vi "4_6.vi"() -> ()   [LabVIEW 2020]
uses:
  <vilib>/numeric/Random Number (Range) U64.vi
  <vilib>/numeric/sub_Random U32.vi
panel:
  in  "Numeric":i32
  out "nieparzyste":u64[](array[numeric])
  out "parzyste":u64[](array[numeric])
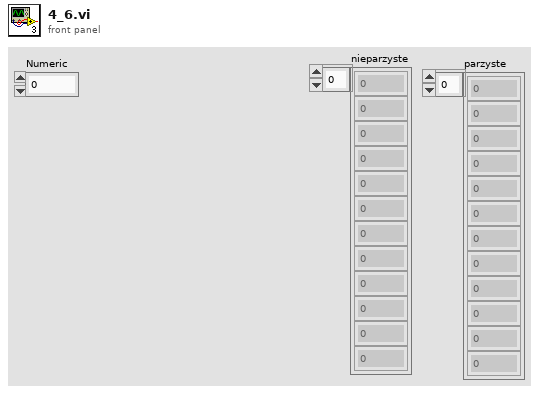
[diagram p1: front panel]
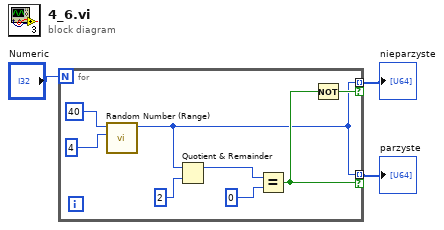
[diagram p0: block diagram]
diagram:
  n1 = for {
    N: "Numeric" -> [_]
    tunnel: [w4] -> w1 mode=indexing if=w5
    tunnel: [w4] -> w3 mode=indexing if=w6
    n2 = call-poly <vilib>:"Random Number (Range).vi"("lower bound (0)"=u64 4, "upper bound (100)"=u64 40) -> ("number"=w4:u64)  [unwired: 9 in]
    n3 = Quotient & Remainder(x=w4, y=u64 2) -> (x-y*floor(x/y)=w8:u64)  [unwired: 1 out]
    n4 = Equal?(x=w8, y=u64 0) -> (x = y?=w5:bool)
    n5 = Not(x=w5) -> (.not. x?=w6:bool)
  }
  "parzyste" <- w1
  "nieparzyste" <- w3
